vi "_ReadExceldata_vna_jet.vi"(2 "sheet":i32=1, 3 "值列":i32, 4 "起始行":i32=4, 5 "路径":path=path "C:/Users/wmg/Desktop/LabelList.xlsx") -> (1 "数据":string[][](array[string])=[["L01HE007-SD-R", "年月日", "16", "16", "", "", "17", "17", "18", "18", "19", "22"], ["L01HE008-SD-R", "年月日", "16", "16", "", "", "17", "17", "18", "18", "19", "22"]])   [LabVIEW 2011]
panel:
  out "Flag":i32=4
  in  "Excel._Worksheet":refnum<k7>
  in  "Excel._Application":refnum<k7>
  # "一行说明+三行例子\n从“4”开始"
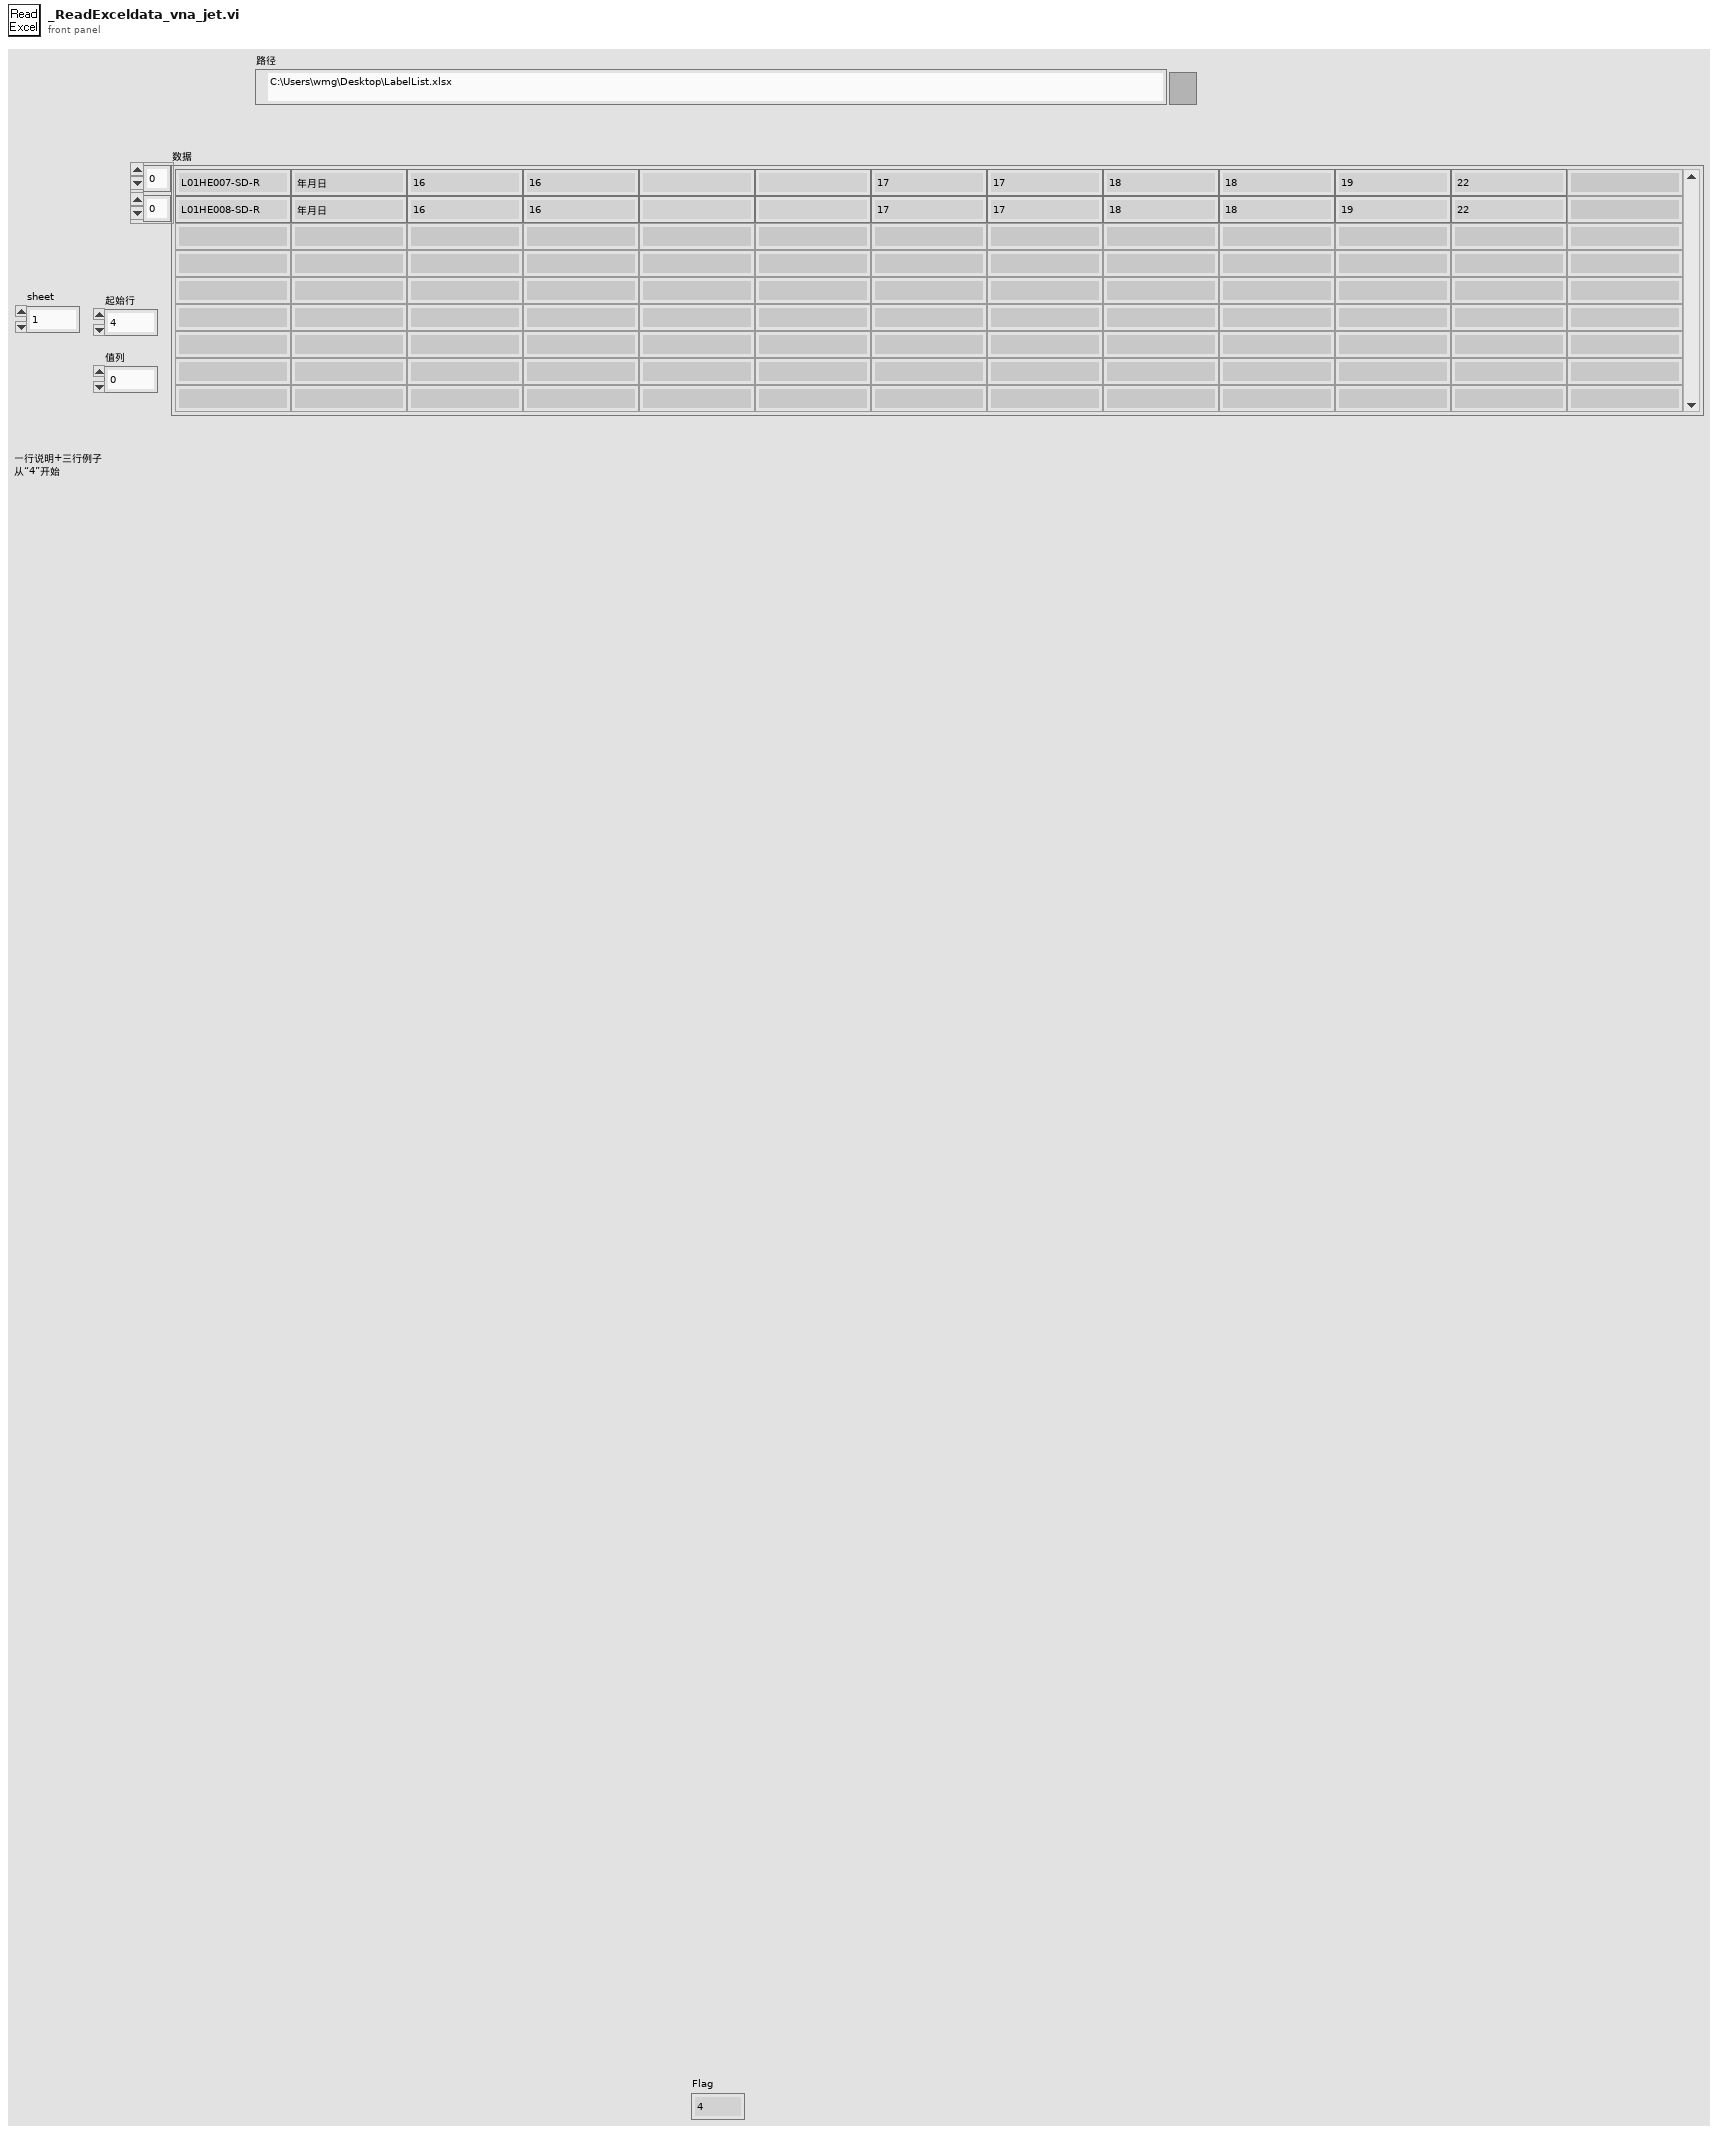
[diagram p1: front panel]
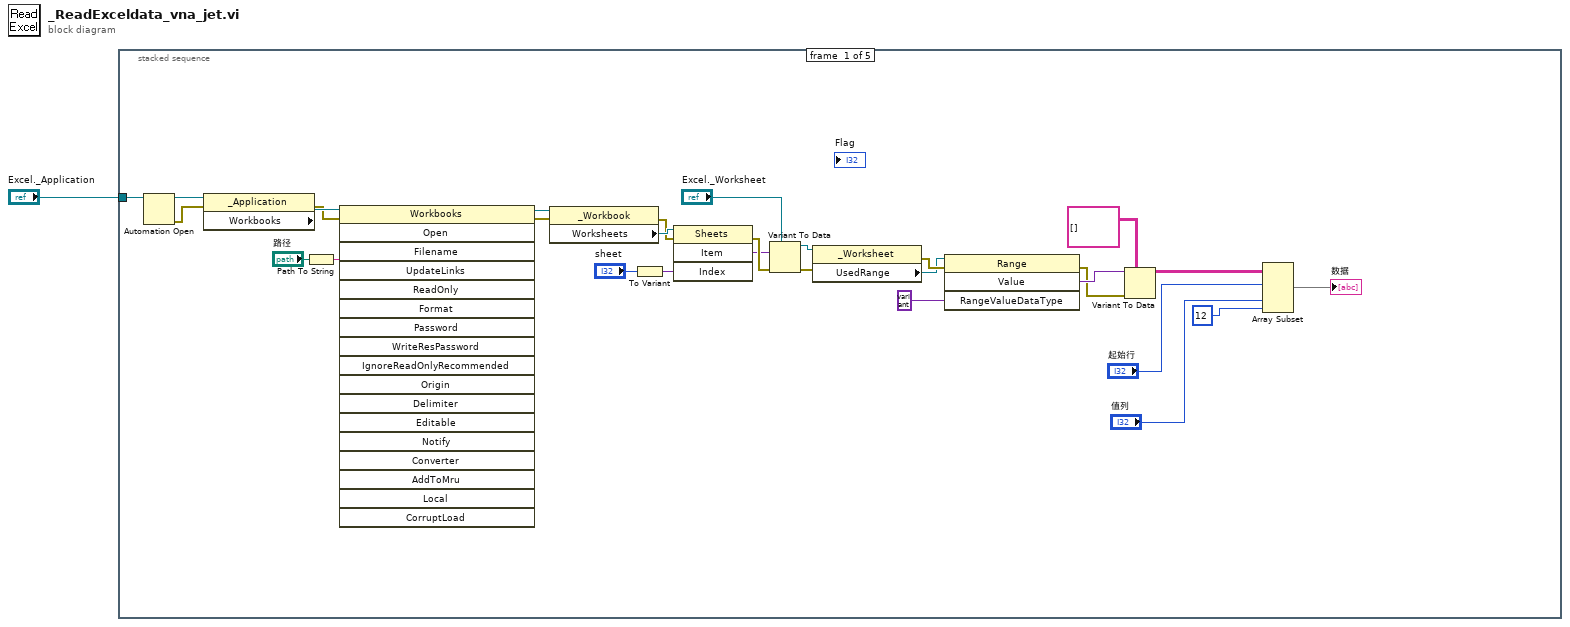
[diagram p0: block diagram]
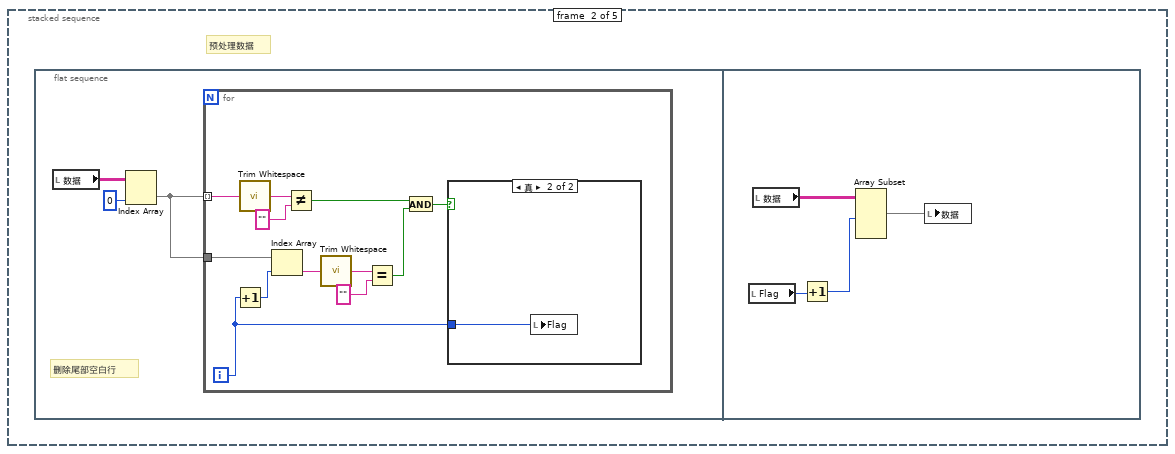
[diagram p2: hidden frame]
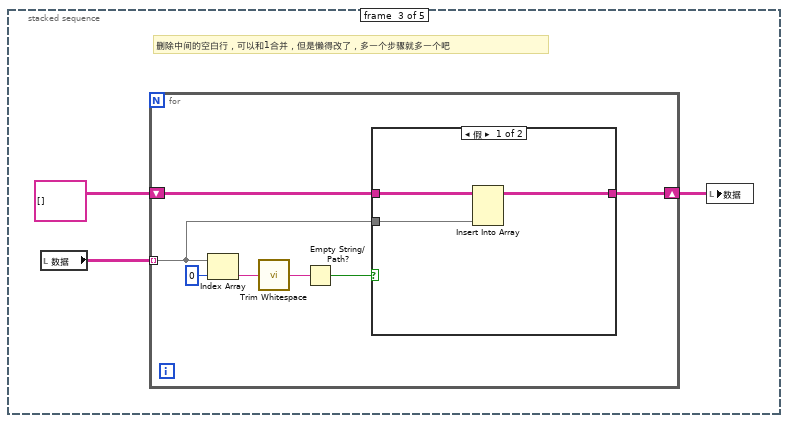
[diagram p4: hidden frame]
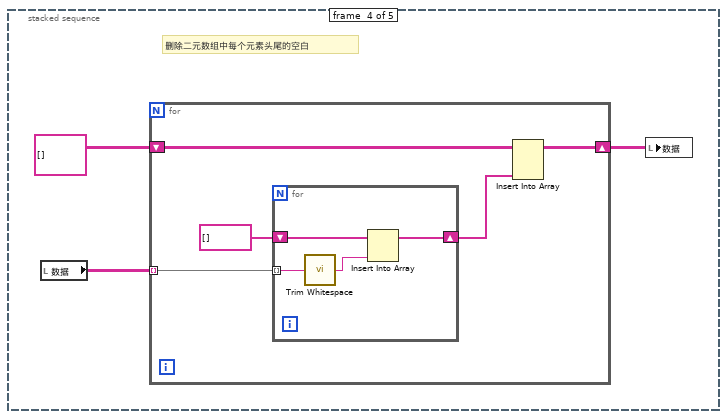
[diagram p6: hidden frame]
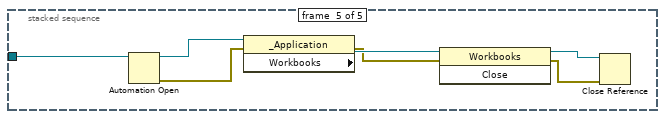
[diagram p7: hidden frame]
diagram:
  n1 = stacked-sequence {
    tunnel: "Excel._Application" -> [w10 _ _ _ w77]
    frame #0 {
      n2 = Automation Open(Automation Refnum=w10) -> (Automation Refnum=w30:refnum<k7>, error out=w29:errorcluster)  [unwired: 3 in]
      n3 = property class="_Application"(reference=w30, error in=w29) -> (error out=w27:errorcluster, "Workbooks"=w28:refnum<k7>)  [unwired: 1 out]
      n4 = Path To String(path="路径") -> (string=w26:string)
      n5 = invoke class="Workbooks" method="Open"(reference=w28, error in=w27, "Filename"=w26) -> (error out=w24:errorcluster, "Open"=w25:refnum<k7>)  [unwired: 15 in, 16 out]
      n6 = property class="_Workbook"(reference=w25, error in=w24) -> (error out=w19:errorcluster, "Worksheets"=w23:refnum<k7>)  [unwired: 1 out]
      n7 = To Variant(anything="sheet") -> (Variant=w21:variant)
      n8 = invoke class="Sheets" method="Item"(reference=w23, error in=w19, "Index"=w21) -> (error out=w20:errorcluster, "Item"=w18:variant)  [unwired: 1 in, 2 out]
      n9 = Variant To Data(error in=w20, type="Excel._Worksheet", Variant=w18) -> (data=w7:refnum<k7>, error out=w16:errorcluster)
      n10 = property class="_Worksheet"(reference=w7, error in=w16) -> (error out=w13:errorcluster, "UsedRange"=w8:refnum<k7>)  [unwired: 1 out]
      n11 = invoke class="Range" method="Value"(reference=w8, error in=w13, "RangeValueDataType"=variant) -> (error out=w11:errorcluster, "Value"=w15:variant)  [unwired: 1 in, 2 out]
      n12 = Variant To Data(error in=w11, type=string[][] [] ("添加的数组"), Variant=w15) -> (data=w6:string[][])  [unwired: 1 out]
      n13 = Array Subset(array=w6, index (row)="起始行", index (col)="值列", length (col)=12) -> (→"数据":string[][])  [unwired: 1 in]
    }
    frame #1 {
      # "预处理数据"
      n14 = flat-sequence {
        frame #0 {
          # "删除尾部空白行"
          n15 = local read "数据"() -> (w33:string[][])
          n16 = Index Array(array=w33, index (col)=0 ("禁用的索引 (列)")) -> (element=w31:string[])  [unwired: 1 in]
          n17 = for {
            tunnel: w31 -> [w43] mode=indexing
            tunnel: w31 -> [w40]
            i -> [w34]
            n18 = Increment(x=w34) -> (x+1=w39:i32)
            n19 = call <vilib>:"Trim Whitespace.vi"("string"=w43) -> ("trimmed string"=w45:string)  [unwired: 1 in]
            n20 = Index Array(array=w40, index=w39) -> (element=w38:string)
            n21 = Not Equal?(x=w45, y="") -> (x != y?=w37:bool)
            n22 = call <vilib>:"Trim Whitespace.vi"("string"=w38) -> ("trimmed string"=w41:string)  [unwired: 1 in]
            n23 = Equal?(x=w41, y="") -> (x = y?=w36:bool)
            n24 = And(x=w37, y=w36) -> (x .and. y?=w35:bool)
            n25 = case shown="真" w35 {
              tunnel: w34 -> [_ w46]
              frame False {
              }
              frame True {
                n26 = local write "Flag"(w46) -> ()
              }
            }
          }
        }
        frame #1 {
          n27 = local read "Flag"() -> (w49:i32)
          n28 = local read "数据"() -> (w50:string[][])
          n29 = Increment(x=w49) -> (x+1=w48:i32)
          n30 = Array Subset(array=w50, length (row)=w48) -> (w47:string[][])  [unwired: 3 in]
          n31 = local write "数据"(w47) -> ()
        }
      }
    }
    frame #2 {
      # "删除中间的空白行，可以和1合并，但是懒得改了，多一个步骤就多一个吧"
      n32 = local read "数据"() -> (w53:string[][])
      n33 = for {
        tunnel: w53 -> [w54] mode=indexing
        shift-right: [w55] -> w51
        shift-left: string[][] [] -> [w56]
        n34 = Index Array(array=w54, index=0 ("索引")) -> (element=w59:string)
        n35 = call <vilib>:"Trim Whitespace.vi"("string"=w59) -> ("trimmed string"=w58:string)  [unwired: 1 in]
        n36 = Empty String/Path?(string/path=w58) -> (empty?=w57:bool)
        n37 = case shown="假" w57 {
          tunnel: w56 -> [w63 w64]
          tunnel: [w62 w64] -> w55
          tunnel: w54 -> [w61 _]
          frame False {
            n38 = Insert Into Array(array=w63, new element=w61) -> (w62:string[][])  [unwired: 2 in]
          }
          frame True {
            # "为空"
          }
        }
      }
      n39 = local write "数据"(w51) -> ()
    }
    frame #3 {
      # "删除二元数组中每个元素头尾的空白"
      n40 = local read "数据"() -> (w67:string[][])
      n41 = for {
        tunnel: w67 -> [w72] mode=indexing
        shift-right: [w69] -> w65
        shift-left: string[][] [] -> [w70]
        n42 = for {
          tunnel: w72 -> [w76] mode=indexing
          shift-right: [w73] -> w68
          shift-left: string[] [] -> [w75]
          n43 = call <vilib>:"Trim Whitespace.vi"("string"=w76) -> ("trimmed string"=w74:string)  [unwired: 1 in]
          n44 = Insert Into Array(array=w75, new element=w74) -> (w73:string[])  [unwired: 1 in]
        }
        n45 = Insert Into Array(array=w70, new element=w68) -> (w69:string[][])  [unwired: 2 in]
      }
      n46 = local write "数据"(w65) -> ()
    }
    frame #4 {
      n47 = Automation Open(Automation Refnum=w77) -> (Automation Refnum=w83:refnum<k7>, error out=w82:errorcluster)  [unwired: 3 in]
      n48 = property class="_Application"(reference=w83, error in=w82) -> (error out=w80:errorcluster, "Workbooks"=w81:refnum<k7>)  [unwired: 1 out]
      n49 = invoke class="Workbooks" method="Close"(reference=w81, error in=w80) -> (reference out=w78:refnum<k7>, error out=w79:errorcluster)  [unwired: 1 in, 1 out]
      n50 = Close Reference(reference=w78, error in (no error)=w79) -> ()  [unwired: 1 out]
    }
  }
